vi "Identify.vi"(0 "reference in":refnum<class "Simulated-PowerModule.lvclass">, 11 "Error In":errorcluster) -> (4 "reference out":refnum<class "Simulated-PowerModule.lvclass">, 6 "identity":string, 15 "Error Out":errorcluster)   [LabVIEW 2023, in "Simulated-PowerModule.lvlib" / "Simulated-PowerModule.lvclass"]
uses:
  Simulated-PowerModule.lvclass
  Simulated-PowerModule.lvclass/Simulated-PowerModule.ctl
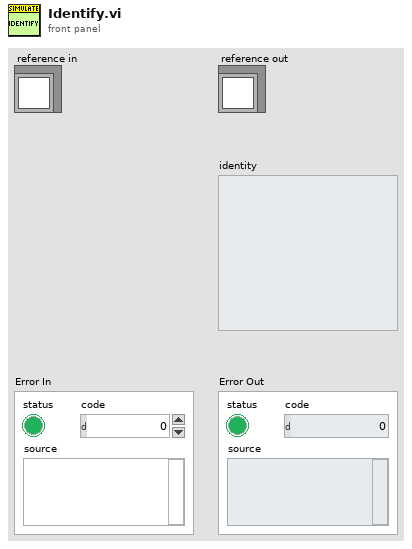
[diagram p1: front panel]
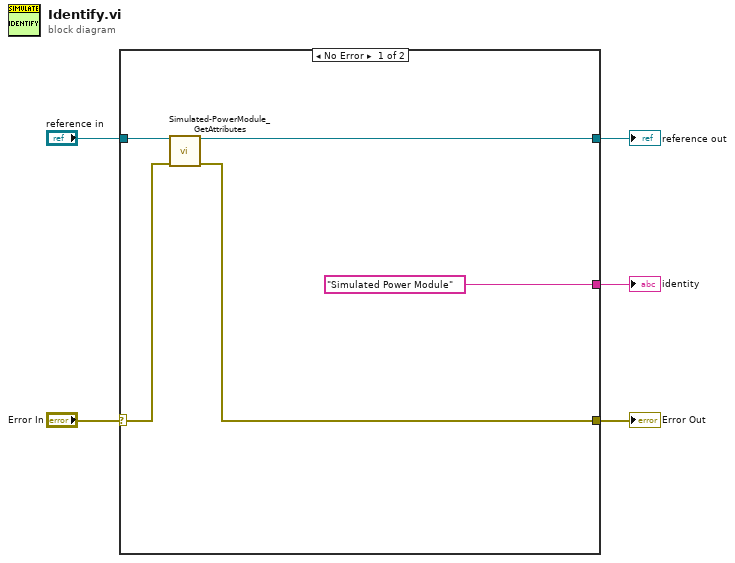
[diagram p0: block diagram]
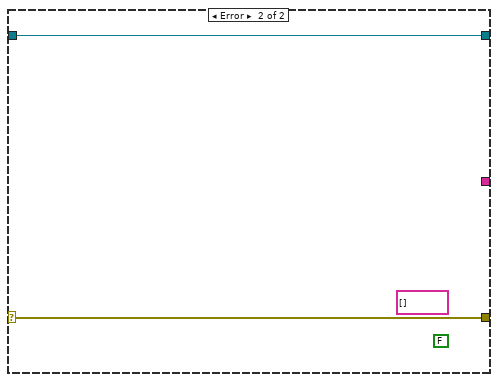
[diagram p2: hidden frame]
diagram:
  n1 = case shown="No Error" "Error In" {
    selector: "Error In" -> [w9 w11]
    tunnel: "reference in" -> [w10 w12]
    tunnel: [w8 w12] -> w3
    tunnel: [w7 w11] -> w2
    tunnel: ["Simulated Power Module" ("JSON String") _] -> w1
    frame No Error {
      n2 = call "Simulated-PowerModule_GetAttributes.vi"("reference in"=w10, "Error In"=w9) -> ("reference out"=w8:refnum<class "Simulated-PowerModule.lvclass">, "Error Out"=w7:errorcluster)  [unwired: 10 in, 2 out]
    }
    frame Error {
      (unwired) string[] []
      (unwired) FALSE
    }
  }
  "Error Out" <- w2
  "reference out" <- w3
  "identity" <- w1
